vi "Set Chamber.vi"(8 "error in (no error)":errorcluster, 10 "Action":string, 11 "Instrument.Cryostat in":refnum<class "Instrument.Cryostat.lvclass">) -> (0 "error out":errorcluster, 3 "Instrument.Cryostat out":refnum<class "Instrument.Cryostat.lvclass">)   [LabVIEW 2019, in "Instrument.Cryostat.lvclass"]
uses:
  Instrument.Cryostat.lvclass
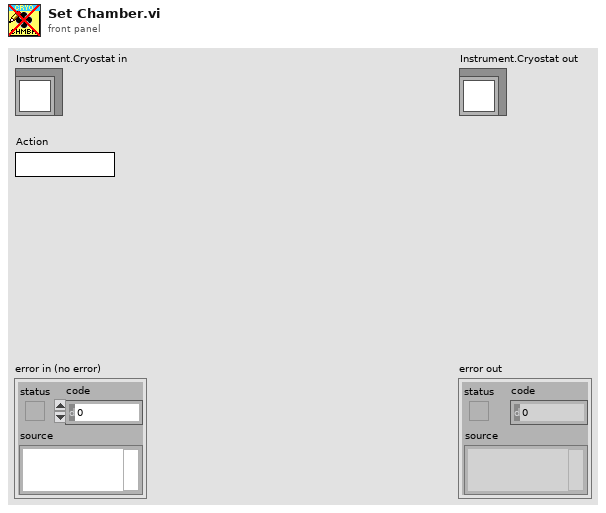
[diagram p1: front panel]
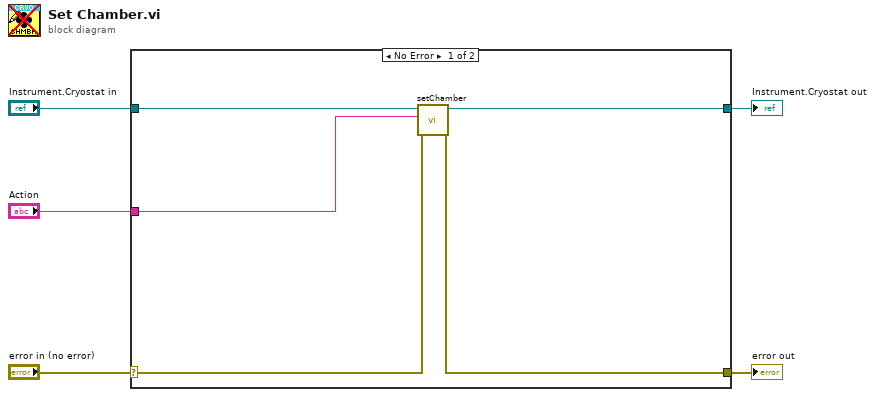
[diagram p0: block diagram]
diagram:
  n1 = case shown="No Error" "error in (no error)" {
    selector: "error in (no error)" -> [w8 w12]
    tunnel: [w7 w12] -> w4
    tunnel: [w10 w11] -> w2
    tunnel: "Instrument.Cryostat in" -> [w9 w11]
    tunnel: "Action" -> [w6 _]
    frame No Error {
      n2 = call-dynamic "setChamber.vi"("error in (no error)"=w8, "Action"=w6, "Instrument.Cryostat in"=w9) -> ("error out"=w7:errorcluster, "Instrument.Cryostat out"=w10:refnum<class "Instrument.Cryostat.lvclass">)  [unwired: 7 in]
    }
    frame Error {
    }
  }
  "error out" <- w4
  "Instrument.Cryostat out" <- w2
